vi "Single Z Ramp Approach Experimental Bundle.vi"() -> (0 "Input Channels":string, 1 "Output Channels":string, 2 "Output Waveforms":waveform(dbl)[](array[waveform]))   [LabVIEW 2013]
uses:
  <vilib>/Waveform/WDTOps.llb/WDT Append Waveforms DBL.vi
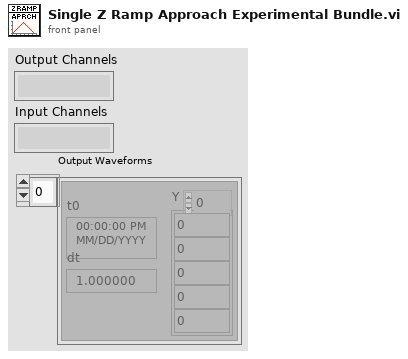
[diagram p1: front panel]
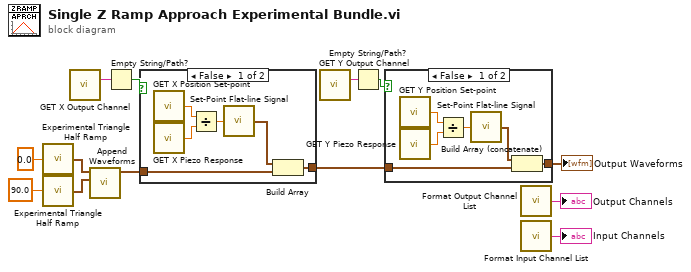
[diagram p0: block diagram]
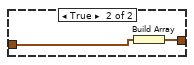
[diagram p3: hidden frame]
diagram:
  n1 = call "Experimental Triangle Half Ramp.vi"("Phase Offset"=0.0) -> ("Half Triangle"=w2:waveform(dbl))
  n2 = call "Experimental Triangle Half Ramp.vi"("Phase Offset"=90.0) -> ("Half Triangle"=w5:waveform(dbl))
  n3 = call "GET X Output Channel.vi"() -> ("X Output Channel"=w10:string)
  n4 = call-poly <vilib>:"Append Waveforms.vi"("waveform B"=w5, "waveform A"=w2) -> ("waveform out"=w1:waveform(dbl))  [unwired: 8 in, 1 out]
  n5 = Empty String/Path?(string/path=w10) -> (empty?=w11:bool)
  n6 = case shown="False" w11 {
    tunnel: w1 -> [w16 w20]
    tunnel: [w14 w21] -> w12
    frame False {
      n7 = call "GET X Position Set-point.vi"() -> ("X Position Set-point"=w18:dbl)
      n8 = call "GET X Piezo Response.vi"() -> ("X Piezo Response"=w19:dbl)
      n9 = Divide(x=w18, y=w19) -> (x/y=w17:dbl)
      n10 = call "Set-Point Flat-line Signal.vi"("Flatline Offset"=w17) -> ("Flatline Signal"=w15:waveform(dbl))
      n11 = Build Array(w15, w16) -> (w14:waveform(dbl)[])
    }
    frame True {
      n12 = Build Array(w20) -> (w21:waveform(dbl)[])
    }
  }
  n13 = call "GET Y Output Channel.vi"() -> ("Y Output Channel"=w8:string)
  n14 = Empty String/Path?(string/path=w8) -> (empty?=w9:bool)
  n15 = case shown="False" w9 {
    tunnel: w12 -> [w24 w28]
    tunnel: [w22 w28] -> w13
    frame False {
      n16 = call "GET Y Position Set-point.vi"() -> ("Y Position Set-point"=w26:dbl)
      n17 = call "GET Y Piezo Response.vi"() -> ("Y Piezo Response"=w27:dbl)
      n18 = Divide(x=w26, y=w27) -> (x/y=w25:dbl)
      n19 = call "Set-Point Flat-line Signal.vi"("Flatline Offset"=w25) -> ("Flatline Signal"=w23:waveform(dbl))
      n20 = Build Array (concatenate)(w23, w24) -> (w22:waveform(dbl)[])
    }
    frame True {
    }
  }
  "Output Waveforms" <- w13
  n21 = call "Format Output Channel List.vi"() -> ("Output Channels"=→"Output Channels":string)
  n22 = call "Format Input Channel List.vi"() -> ("Input Channels"=→"Input Channels":string)
